vi "SpoolToDisk.vi"() -> ()   [LabVIEW 2009]
uses:
  <vilib>/Utility/importsl/GetValueByPointer/GetValueByPointer.xnode
  <vilib>/Utility/importsl/GetValueByPointer/datatype.ctl
  resource/lvimptsl.dll
panel:
  in  "Pixel Readout Rate":string(combo)
  in  "Overlap":bool
  in  "Shutter":string(combo)
  out "FrameRate":dbl
  out "Current Image":i32
  in  "Path":path
  in  "NumImages":i32
  in  "Centre AOI":bool
  in  "AOI Width":i64
  in  "AOI Height":i64
  out "Ready":bool
  in  "Run":bool
  in  "error":errorcluster
  out "Pixel Encoding":string
  out "AOIStride":i64
  in  "PreAmp":string(combo)
  out "PixelData":u16[](array[numeric])
  out "ByteData":u8[](array[numeric])
  in  "ExposureTime":dbl
  out "ImageSizeBytes":i64
  out "Handle":i32
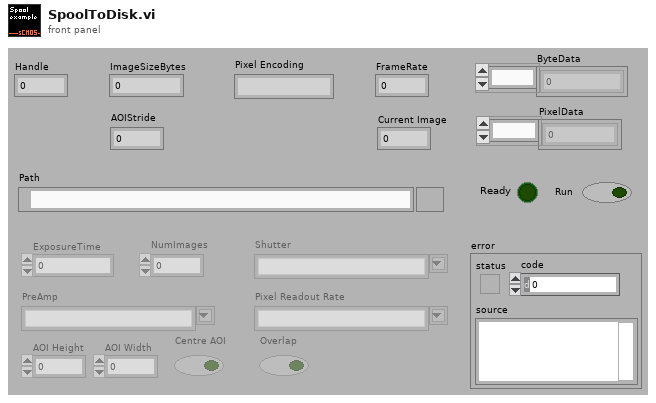
[diagram p1: front panel]
types:
  T1 = enum8{"Enabled", "Disabled", "Disabled and Grayed Out"}
  T2 = enum16{"big-endian, network order", "native, host order", "little-endian"}
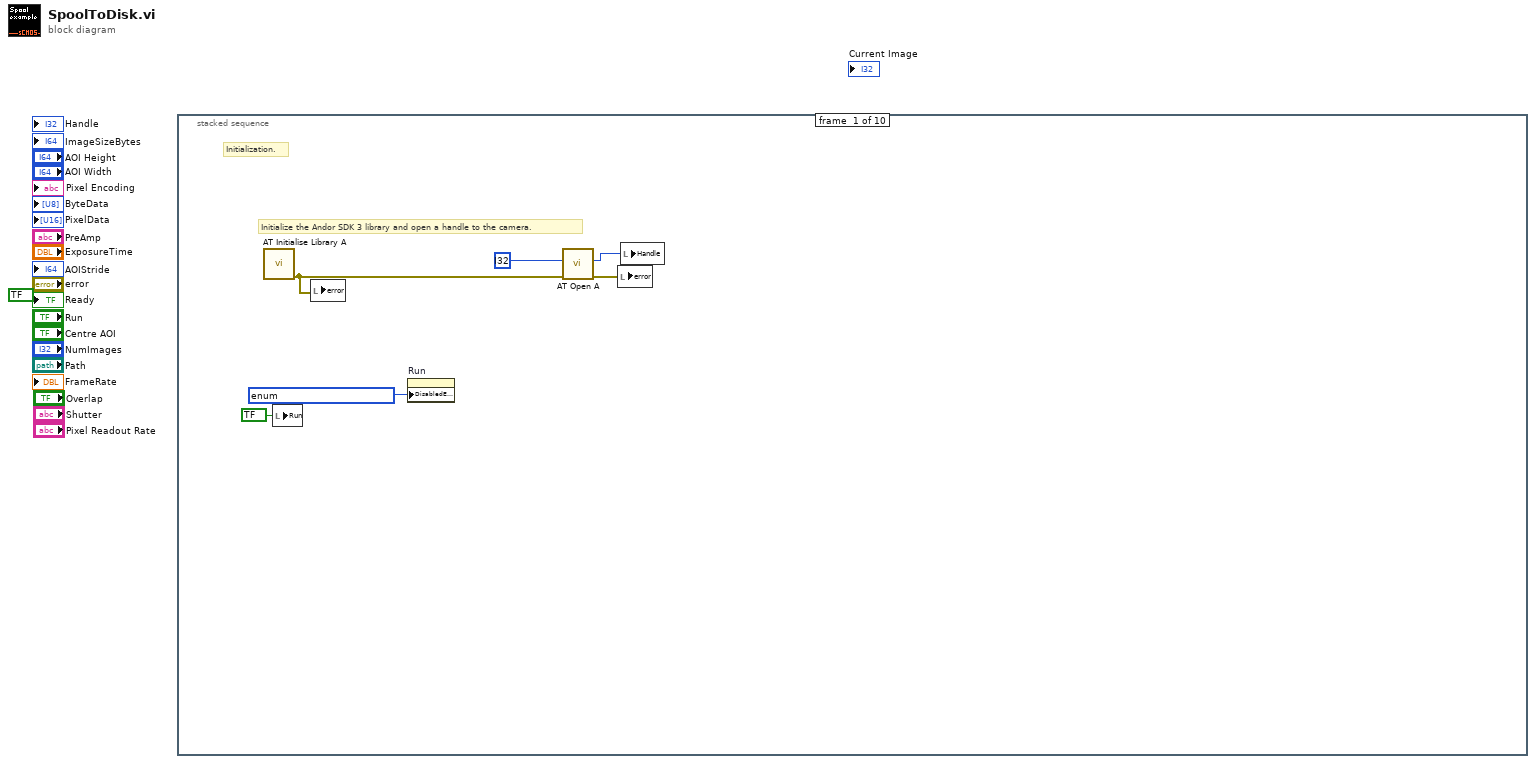
[diagram p0: block diagram]
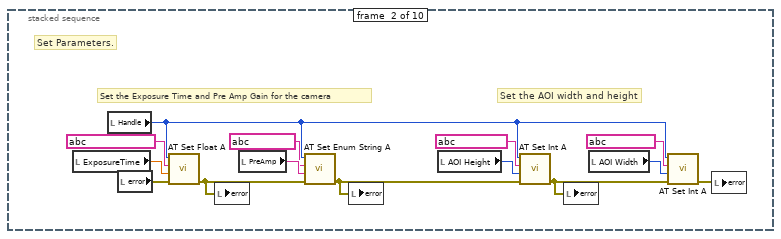
[diagram p2: hidden frame]
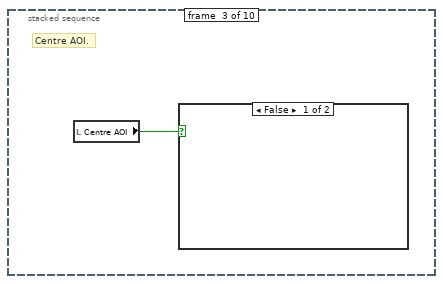
[diagram p3: hidden frame]
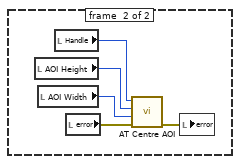
[diagram p4: hidden frame]
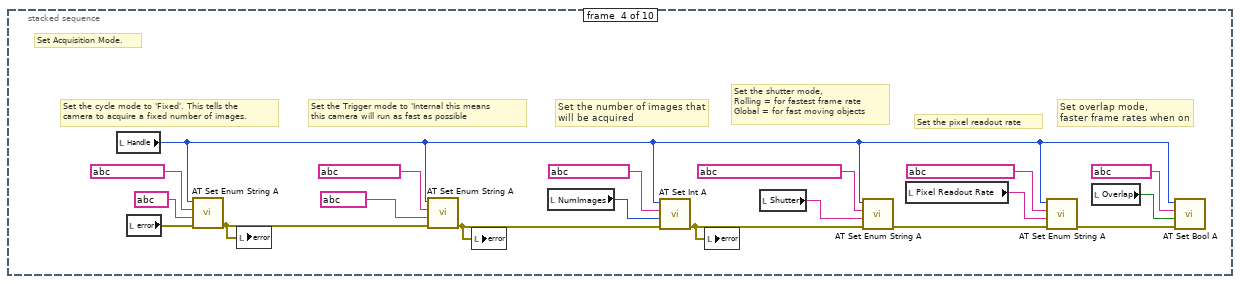
[diagram p5: hidden frame]
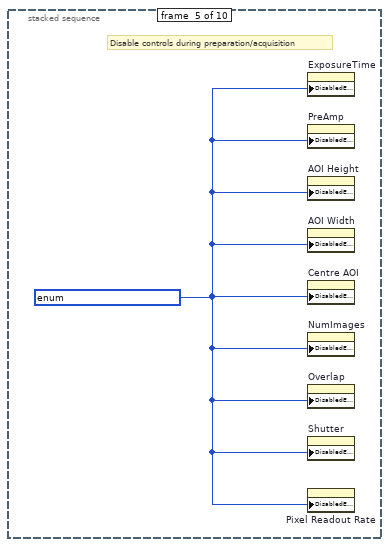
[diagram p6: hidden frame]
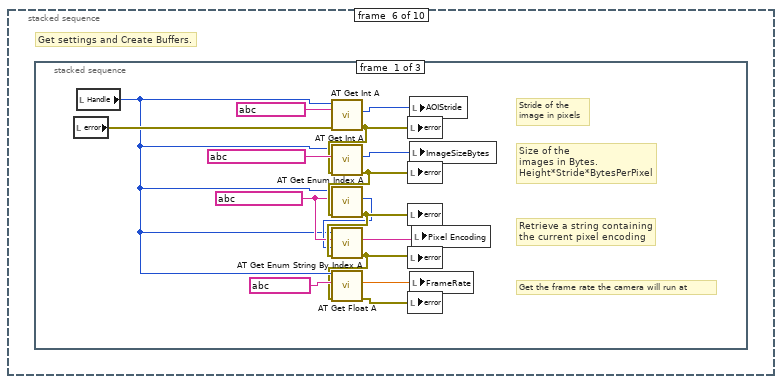
[diagram p7: hidden frame]
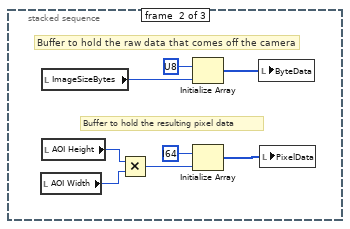
[diagram p8: hidden frame]
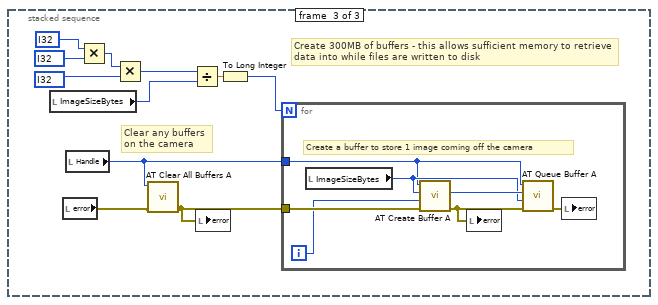
[diagram p9: hidden frame]
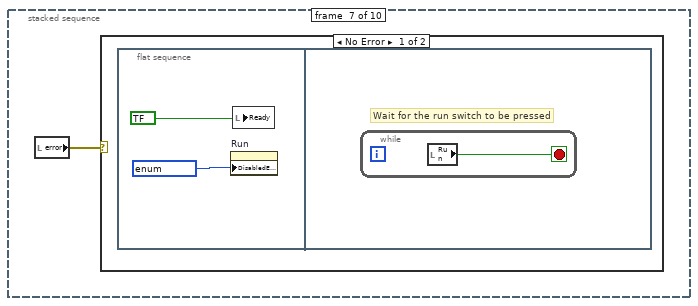
[diagram p10: hidden frame]
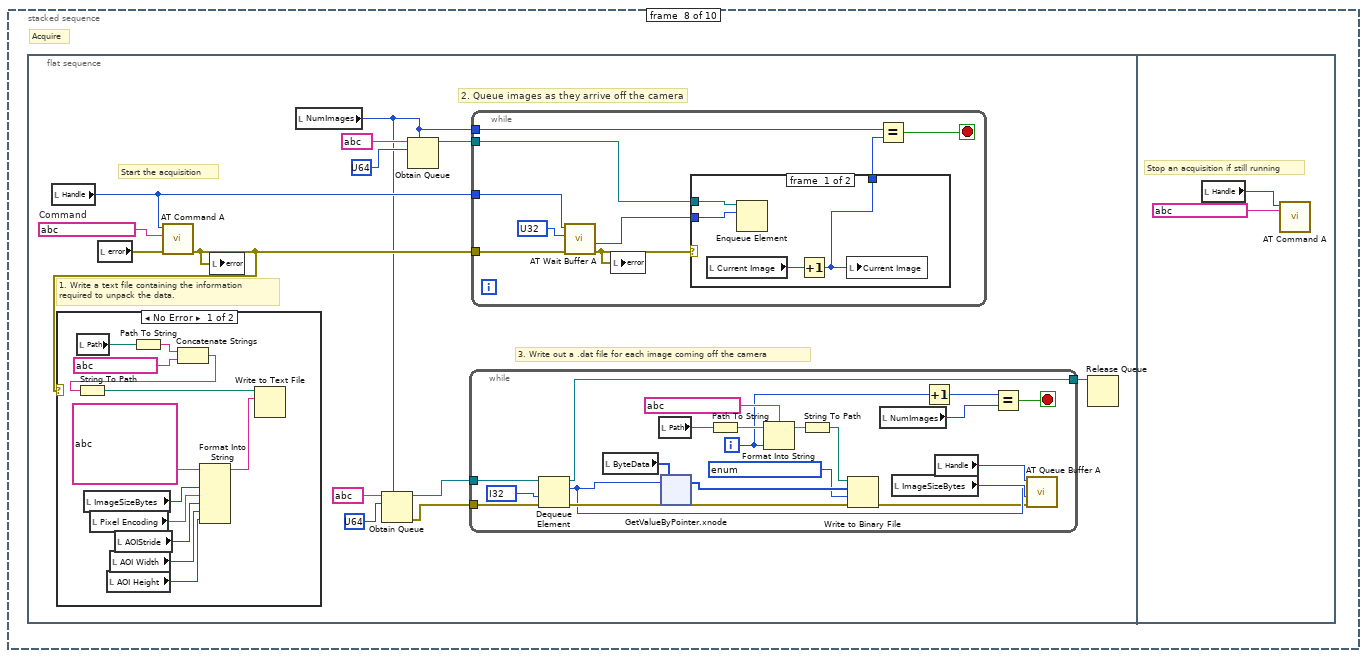
[diagram p12: hidden frame]
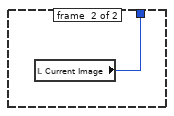
[diagram p13: hidden frame]
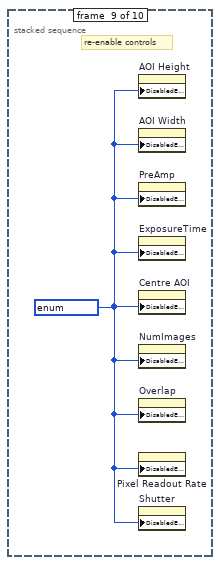
[diagram p15: hidden frame]
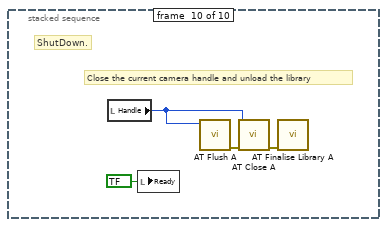
[diagram p16: hidden frame]
diagram:
  n1 = stacked-sequence {
    frame #0 {
      # "Initialize the Andor SDK 3 library and open a handle to the camera."
      # "Initialization."
      n2 = call "AT Initialise Library A.vi"() -> ("error out"=w3:errorcluster)  [unwired: 10 in, 1 out]
      n3 = local write "Run"(bool ? ("Run")) -> ()
      n4 = local write "error"(w3) -> ()
      n5 = property on="Run" class="Bool (strict)"("DisabledEnum"=T1 ? ("Disabled")) -> ()  [unwired: 2 in, 2 out]
      n6 = call "AT Open A.vi"("error in (no error)"=w3, "CameraIndex"=i32 ?) -> ("error out"=w2:errorcluster, "Handle"=w4:i32)  [unwired: 7 in, 1 out]
      n7 = local write "error"(w2) -> ()
      n8 = local write "Handle"(w4) -> ()
    }
    frame #1 {
      # "Set the AOI width and height"
      # "Set the Exposure Time and Pre Amp Gain for the camera"
      # "Set Parameters."
      n9 = local read "ExposureTime"() -> (w21:dbl)
      n10 = local read "Handle"() -> (w8:i32)
      n11 = local read "error"() -> (w16:errorcluster)
      n12 = call "AT Set Float A.vi"("error in (no error)"=w16, "Value"=w21, "Feature"=string ? ("ExposureTime"), "Hndl"=w8) -> ("error out"=w19:errorcluster)  [unwired: 6 in, 1 out]
      n13 = local write "error"(w19) -> ()
      n14 = local read "PreAmp"() -> (w20:string)
      n15 = call "AT Set Enum String A.vi"("error in (no error)"=w19, "String"=w20, "Feature"=string ? ("SimplePreAmpGainControl"), "Handle"=w8) -> ("error out"=w15:errorcluster)  [unwired: 6 in, 1 out]
      n16 = local write "error"(w15) -> ()
      n17 = local read "AOI Height"() -> (w12:i64)
      n18 = call "AT Set Int A.vi"("error in (no error)"=w15, "Value"=w12, "Feature"=string ? ("Integer feature"), "Handle"=w8) -> ("error out"=w13:errorcluster)  [unwired: 6 in, 1 out]
      n19 = local write "error"(w13) -> ()
      n20 = local read "AOI Width"() -> (w11:i64)
      n21 = call "AT Set Int A.vi"("error in (no error)"=w13, "Value"=w11, "Feature"=string ? ("Integer feature 2"), "Handle"=w8) -> ("error out"=w14:errorcluster)  [unwired: 6 in, 1 out]
      n22 = local write "error"(w14) -> ()
    }
    frame #2 {
      # "Centre AOI."
      n23 = local read "Centre AOI"() -> (w22:bool)
      n24 = case shown="False" w22 {
        frame #0 {
        }
        frame #1 {
          n25 = local read "AOI Height"() -> (w24:i64)
          n26 = local read "AOI Width"() -> (w25:i64)
          n27 = local read "Handle"() -> (w23:i32)
          n28 = local read "error"() -> (w26:errorcluster)
          n29 = call "AT Centre AOI.vi"("error in (no error)"=w26, "AOI Width"=w25, "AOI Height"=w24, "Handle"=w23) -> ("error out"=w27:errorcluster)  [unwired: 7 in]
          n30 = local write "error"(w27) -> ()
        }
      }
    }
    frame #3 {
      # "Set overlap mode,\nfaster frame rates when on"
      # "Set the pixel readout rate"
      # "Set the shutter mode,\nRolling = for fastest frame rate\nGlobal = for fast moving objects"
      # "Set the number of images that \nwill be acquired"
      # "Set the Trigger mode to 'Internal this means \nthis camera will run as fast as possible"
      # "Set the cycle mode to 'Fixed'. This tells the \ncamera to acquire a fixed number of images."
      # "Set Acquisition Mode."
      n31 = local read "Handle"() -> (w33:i32)
      n32 = local read "error"() -> (w44:errorcluster)
      n33 = call "AT Set Enum String A.vi"("error in (no error)"=w44, "String"=string ?, "Feature"=string ? ("Enum feature"), "Handle"=w33) -> ("error out"=w43:errorcluster)  [unwired: 6 in, 1 out]
      n34 = local write "error"(w43) -> ()
      n35 = call "AT Set Enum String A.vi"("error in (no error)"=w43, "String"=string ?, "Feature"=string ? ("Enum feature"), "Handle"=w33) -> ("error out"=w40:errorcluster)  [unwired: 6 in, 1 out]
      n36 = local write "error"(w40) -> ()
      n37 = local read "NumImages"() -> (w38:i32)
      n38 = call "AT Set Int A.vi"("error in (no error)"=w40, "Value"=w38, "Feature"=string ? ("Integer feature 2"), "Handle"=w33) -> ("error out"=w37:errorcluster)  [unwired: 6 in, 1 out]
      n39 = local write "error"(w37) -> ()
      n40 = local read "Shutter"() -> (w30:string)
      n41 = call "AT Set Enum String A.vi"("error in (no error)"=w37, "String"=w30, "Feature"=string ? ("ElectronicShutteringMode"), "Handle"=w33) -> ("error out"=w36:errorcluster)  [unwired: 6 in, 1 out]
      n42 = local read "Pixel Readout Rate"() -> (w29:string)
      n43 = call "AT Set Enum String A.vi"("error in (no error)"=w36, "String"=w29, "Feature"=string ? ("PixelReadoutRate"), "Handle"=w33) -> ("error out"=w35:errorcluster)  [unwired: 6 in, 1 out]
      n44 = local read "Overlap"() -> (w28:bool)
      n45 = call "AT Set Bool A.vi"("error in (no error)"=w35, "Value"=w28, "Feature"=string ? ("Overlap"), "Handle"=w33) -> ()  [unwired: 6 in, 2 out]
    }
    frame #4 {
      w47 = T1 ? ("Disabled")
      # "Disable controls during preparation/acquisition"
      n46 = property on="ExposureTime" class="DigNum (strict)"("DisabledEnum"=w47) -> ()  [unwired: 2 in, 2 out]
      n47 = property on="PreAmp" class="CmbBox"("DisabledEnum"=w47) -> ()  [unwired: 2 in, 2 out]
      n48 = property on="AOI Height" class="DigNum (strict)"("DisabledEnum"=w47) -> ()  [unwired: 2 in, 2 out]
      n49 = property on="AOI Width" class="DigNum (strict)"("DisabledEnum"=w47) -> ()  [unwired: 2 in, 2 out]
      n50 = property on="Centre AOI" class="Bool (strict)"("DisabledEnum"=w47) -> ()  [unwired: 2 in, 2 out]
      n51 = property on="NumImages" class="DigNum (strict)"("DisabledEnum"=w47) -> ()  [unwired: 2 in, 2 out]
      n52 = property on="Overlap" class="Bool (strict)"("DisabledEnum"=w47) -> ()  [unwired: 2 in, 2 out]
      n53 = property on="Shutter" class="CmbBox"("DisabledEnum"=w47) -> ()  [unwired: 2 in, 2 out]
      n54 = property on="Pixel Readout Rate" class="CmbBox"("DisabledEnum"=w47) -> ()  [unwired: 2 in, 2 out]
    }
    frame #5 {
      # "Get settings and Create Buffers."
      n55 = stacked-sequence {
        frame #0 {
          w56 = string ? ("Enum feature")
          # "Get the frame rate the camera will run at"
          # "Retrieve a string containing \nthe current pixel encoding"
          # "Stride of the\nimage in pixels"
          # "Size of the\nimages in Bytes.\nHeight*Stride*BytesPerPixel"
          n56 = local read "error"() -> (w53:errorcluster)
          n57 = local read "Handle"() -> (w50:i32)
          n58 = call "AT Get Int A.vi"("error in (no error)"=w53, "Feature"=string ? ("Integer feature"), "Handle"=w50) -> ("error out"=w59:errorcluster, "Value"=w63:i64)  [unwired: 6 in, 1 out]
          n59 = call "AT Get Int A.vi"("error in (no error)"=w59, "Feature"=string ? ("Integer feature"), "Handle"=w50) -> ("error out"=w58:errorcluster, "Value"=w62:i64)  [unwired: 6 in, 1 out]
          n60 = call "AT Get Enum Index A.vi"("error in (no error)"=w58, "Feature"=w56, "Handle"=w50) -> ("error out"=w57:errorcluster, "Value"=w55:i32)  [unwired: 6 in, 1 out]
          n61 = call "AT Get Enum String By Index A.vi"("error in (no error)"=w57, "Index"=w55, "Feature"=w56, "Handle"=w50) -> ("error out"=w49:errorcluster, "String"=w54:string)  [unwired: 5 in, 1 out]
          n62 = call "AT Get Float A.vi"("error in (no error)"=w49, "Feature"=string ?, "Handle"=w50) -> ("error out"=w51:errorcluster, "Value"=w48:dbl)  [unwired: 6 in, 1 out]
          n63 = local write "error"(w59) -> ()
          n64 = local write "error"(w58) -> ()
          n65 = local write "error"(w57) -> ()
          n66 = local write "error"(w49) -> ()
          n67 = local write "error"(w51) -> ()
          n68 = local write "AOIStride"(w63) -> ()
          n69 = local write "ImageSizeBytes"(w62) -> ()
          n70 = local write "FrameRate"(w48) -> ()
          n71 = local write "Pixel Encoding"(w54) -> ()
        }
        frame #1 {
          # "Buffer to hold the resulting pixel data"
          # "Buffer to hold the raw data that comes off the camera"
          n72 = local read "AOI Width"() -> (w70:i64)
          n73 = local read "ImageSizeBytes"() -> (w65:i64)
          n74 = local read "AOI Height"() -> (w69:i64)
          n75 = Multiply(x=w69, y=w70) -> (x*y=w64:i64)
          n76 = Initialize Array(u8 ?, w65) -> (w67:u8[])
          n77 = Initialize Array(i64 ?, w64) -> (w68:i64[])
          n78 = local write "ByteData"(w67) -> ()
          n79 = local write "PixelData"(w68) -> ()
        }
        frame #2 {
          # "Create 300MB of buffers - this allows sufficient memory to retrieve \ndata into while files are written to disk"
          # "Clear any buffers \non the camera"
          n80 = local read "ImageSizeBytes"() -> (w75:i64)
          n81 = local read "error"() -> (w82:errorcluster)
          n82 = local read "Handle"() -> (w80:i32)
          n83 = Multiply(x=i32 ?, y=i32 ?) -> (x*y=w78:i32)
          n84 = Multiply(x=w78, y=i32 ?) -> (x*y=w74:i32)
          n85 = call "AT Clear All Buffers A.vi"("error in (no error)"=w82, "Handle"=w80) -> ("error out"=w81:errorcluster)  [unwired: 8 in, 1 out]
          n86 = Divide(x=w74, y=w75) -> (x/y=w73:dbl)
          n87 = local write "error"(w81) -> ()
          n88 = To Long Integer(number=w73) -> (32bit integer=w72:i32)
          n89 = for {
            N: w72 -> [_]
            tunnel: w81 -> [w85]
            tunnel: w80 -> [w84]
            i -> [w83]
            # "Create a buffer to store 1 image coming off the camera"
            n90 = local read "ImageSizeBytes"() -> (w87:i64)
            n91 = call "AT Create Buffer A.vi"("error in (no error)"=w85, "Buffer"=w83, "Size"=w87, "Handle"=w84) -> ("error out"=w88:errorcluster, "Buffer out"=w89:u64)  [unwired: 5 in, 1 out]
            n92 = local write "error"(w88) -> ()
            n93 = call "AT Queue Buffer A.vi"("error in (no error)"=w88, "PtrSize"=w87, "Ptr"=w89, "Handle"=w84) -> ("error out"=w86:errorcluster)  [unwired: 6 in, 1 out]
            n94 = local write "error"(w86) -> ()
          }
        }
      }
    }
    frame #6 {
      n95 = local read "error"() -> (w90:errorcluster)
      n96 = case shown="No Error" w90 {
        frame #0 {
          n97 = flat-sequence {
            frame #0 {
              n98 = property on="Run" class="Bool (strict)"("DisabledEnum"=T1 ? ("Disabled")) -> ()  [unwired: 2 in, 2 out]
              n99 = local write "Ready"(bool ? ("Ready")) -> ()
            }
            frame #1 {
              # "Wait for the run switch to be pressed"
              n100 = while {
                stop <- w93 stop-if-true
                n101 = local read "Run"() -> (w93:bool)
              }
            }
          }
        }
        frame #1 {
        }
      }
    }
    frame #7 {
      # "Acquire"
      n102 = flat-sequence {
        frame #0 {
          w104 = string ?  # Command
          # "2. Queue images as they arrive off the camera"
          # "3. Write out a .dat file for each image coming off the camera"
          # "1. Write a text file containing the information \nrequired to unpack the data."
          # "Start the acquisition"
          n103 = local read "Handle"() -> (w106:i32)
          n104 = local read "error"() -> (w105:errorcluster)
          n105 = call "AT Command A.vi"("error in (no error)"=w105, "Feature"=w104, "Handle"=w106) -> ("error out"=w95:errorcluster)  [unwired: 7 in, 1 out]
          n106 = case shown="No Error" w95 {
            frame #0 {
              n107 = local read "Path"() -> (w132:path)
              n108 = local read "ImageSizeBytes"() -> (w121:i64)
              n109 = local read "Pixel Encoding"() -> (w122:string)
              n110 = local read "AOI Height"() -> (w125:i64)
              n111 = local read "AOI Width"() -> (w124:i64)
              n112 = local read "AOIStride"() -> (w123:i64)
              n113 = Path To String(path=w132) -> (string=w130:string)
              n114 = Concatenate Strings(w130, string ? ("format string")) -> (w129:string)
              n115 = String To Path(string=w129) -> (path=w128:path)
              n116 = Format Into String(format string=string ?, w121, w122, w123, w124, w125) -> (resulting string=w126:string)  [unwired: 2 in, 1 out]
              n117 = Write to Text File(file (use dialog)=w128, text=w126) -> ()  [unwired: 2 in, 3 out]
            }
            frame #1 {
            }
          }
          n118 = local write "error"(w95) -> ()
          n119 = local read "NumImages"() -> (w94:i32)
          n120 = Obtain Queue(max queue size (-1, unlimited)=w94, name (unnamed)=string ?, element data type=u64 ?) -> (queue out=w99:refnum<queue>, error out=w100:errorcluster)  [unwired: 2 in, 1 out]
          n121 = Obtain Queue(max queue size (-1, unlimited)=w94, name (unnamed)=string ?, element data type=u64 ?) -> (queue out=w102:refnum<queue>)  [unwired: 2 in, 2 out]
          n122 = while {
            tunnel: w100 -> [w154]
            tunnel: w99 -> [w153]
            tunnel: [w142] -> w96
            i -> [w135]
            stop <- w141 stop-if-true
            n123 = Dequeue Element(queue=w153, timeout in ms (-1)=i32 ?, error in (no error)=w154) -> (queue out=w142:refnum<queue>, element=w143:u64, error out=w146:errorcluster)  [unwired: 1 out]
            n124 = local read "ByteData"() -> (w147:u8[])
            n125 = local read "Path"() -> (w151:path)
            n126 = xnode "GetValueByPointer.xnode"("Pointer"=w143, "InputType"=w147, "ErrorIn"=w146) -> ("Output"=w139:u8[], "ErrorOut"=w138:errorcluster)  [unwired: 1 in]
            n127 = Path To String(path=w151) -> (string=w148:string)
            n128 = Format Into String(format string=string ?, initial string=w148, w135) -> (resulting string=w149:string)  [unwired: 1 in, 1 out]
            n129 = String To Path(string=w149) -> (path=w140:path)
            n130 = Write to Binary File(file (use dialog)=w140, data=w139, error in=w138, 9:T2 ? ("byte order (0:big-endian, network order)")) -> (error out=w136:errorcluster)  [unwired: 2 in, 2 out]
            n131 = local read "NumImages"() -> (w133:i32)
            n132 = local read "ImageSizeBytes"() -> (w145:i64)
            n133 = Increment(x=w135) -> (x+1=w134:i32)
            n134 = local read "Handle"() -> (w144:i32)
            n135 = Equal?(x=w134, y=w133) -> (x = y?=w141:bool)
            n136 = call "AT Queue Buffer A.vi"("error in (no error)"=w136, "PtrSize"=w145, "Ptr"=w143, "Handle"=w144) -> ()  [unwired: 6 in, 2 out]
          }
          n137 = while {
            tunnel: w106 -> [w114]
            tunnel: w95 -> [w113]
            tunnel: w102 -> [w112]
            tunnel: w94 -> [w108]
            stop <- w107 stop-if-true
            n138 = call "AT Wait Buffer A.vi"("error in (no error)"=w113, "Timeout"=u32 ?, "Handle"=w114) -> ("error out"=w110:errorcluster, "Output buffer"=w111:u64)  [unwired: 5 in, 2 out]
            n139 = local write "error"(w110) -> ()
            n140 = case shown="Error" w110 {
              tunnel: w112 -> [w119 _]
              tunnel: w111 -> [w118 _]
              tunnel: [w116 w120] -> w109
              frame #0 {
                n141 = local read "Current Image"() -> (w117:i32)
                n142 = Enqueue Element(queue=w119, element=w118) -> ()  [unwired: 2 in, 3 out]
                n143 = Increment(x=w117) -> (x+1=w116:i32)
                n144 = local write "Current Image"(w116) -> ()
              }
              frame #1 {
                n145 = local read "Current Image"() -> (w120:i32)
              }
            }
            n146 = Equal?(x=w108, y=w109) -> (x = y?=w107:bool)
          }
          n147 = Release Queue(queue=w96) -> ()  [unwired: 2 in, 3 out]
        }
        frame #1 {
          # "Stop an acquisition if still running"
          n148 = local read "Handle"() -> (w167:i32)
          n149 = call "AT Command A.vi"("Feature"=string ? ("Command"), "Handle"=w167) -> ()  [unwired: 8 in, 2 out]
        }
      }
    }
    frame #8 {
      w168 = T1 ? ("Disabled")
      # "re-enable controls"
      n150 = property on="AOI Height" class="DigNum (strict)"("DisabledEnum"=w168) -> ()  [unwired: 2 in, 2 out]
      n151 = property on="AOI Width" class="DigNum (strict)"("DisabledEnum"=w168) -> ()  [unwired: 2 in, 2 out]
      n152 = property on="PreAmp" class="CmbBox"("DisabledEnum"=w168) -> ()  [unwired: 2 in, 2 out]
      n153 = property on="ExposureTime" class="DigNum (strict)"("DisabledEnum"=w168) -> ()  [unwired: 2 in, 2 out]
      n154 = property on="Centre AOI" class="Bool (strict)"("DisabledEnum"=w168) -> ()  [unwired: 2 in, 2 out]
      n155 = property on="NumImages" class="DigNum (strict)"("DisabledEnum"=w168) -> ()  [unwired: 2 in, 2 out]
      n156 = property on="Overlap" class="Bool (strict)"("DisabledEnum"=w168) -> ()  [unwired: 2 in, 2 out]
      n157 = property on="Pixel Readout Rate" class="CmbBox"("DisabledEnum"=w168) -> ()  [unwired: 2 in, 2 out]
      n158 = property on="Shutter" class="CmbBox"("DisabledEnum"=w168) -> ()  [unwired: 2 in, 2 out]
    }
    frame #9 {
      # "Close the current camera handle and unload the library"
      # "ShutDown."
      n159 = local read "Handle"() -> (w171:i32)
      n160 = local write "Ready"(bool ? ("Ready")) -> ()
      n161 = call "AT Flush A.vi"("Handle"=w171) -> ("error out"=w170:errorcluster)  [unwired: 9 in, 1 out]
      n162 = call "AT Close A.vi"("error in (no error)"=w170, "Handle"=w171) -> ("error out"=w169:errorcluster)  [unwired: 8 in, 1 out]
      n163 = call "AT Finalise Library A.vi"("error in (no error)"=w169) -> ()  [unwired: 9 in, 2 out]
    }
  }
  "Ready" <- bool ? ("Ready")
